vi "Init Msg Self.vi"(6 "Actor Msgs":refnum<class "Msg.lvclass">[](array[class]), 9 "Post-Setup Msgs":refnum<class "Msg.lvclass">[](array[class]), 10 "Pre-Setup Msgs":refnum<class "Msg.lvclass">[](array[class])) -> (3 "Base Msg Self out":refnum<class "Base Msg Self.lvclass">)   [LabVIEW 2020, in "jettl.lvlib" / "Base Msg Self.lvlib" / "Base Msg Self.lvclass"]
uses:
  Base Msg Self.lvclass
  Msg/Msg.lvclass
  Base Msg Self.lvclass/Base Msg Self.ctl
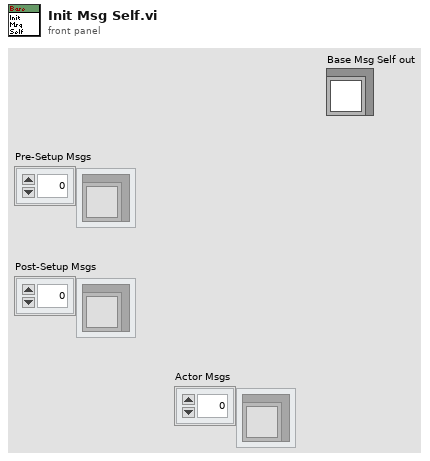
[diagram p1: front panel]
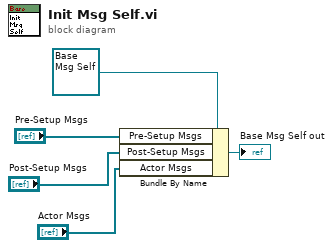
[diagram p0: block diagram]
diagram:
  n1 = Bundle By Name(cluster=refnum<class "Base Msg Self.lvclass"> refnum ("Base Msg Self"), "Pre-Setup Msgs"="Pre-Setup Msgs", "Post-Setup Msgs"="Post-Setup Msgs", "Actor Msgs"="Actor Msgs") -> (→"Base Msg Self out":refnum<class "Base Msg Self.lvclass">)
